vi "AMB_Control.vi"(0 "ObjHandle in":u32, 1 "Data in":u8[](array[numeric]) format="%.0x", 2 "CAN ID in":u32 format="%.0x", 3 "error in":errorcluster {"code" format="%.0x"}, 4 "Data Length in":u8) -> (5 "ObjHandle out":u32, 6 "error out":errorcluster {"code" format="%.0x"})   [LabVIEW 2017]
doc: "ALMA M&C Bus transmit control message\nTransmits a CAN message to the specified ID.\nreally its just a wrapper for the NICAN WriteNet vi."
panel:
  # "ALMA Monitor and Control Bus\nTransmit Control Message"
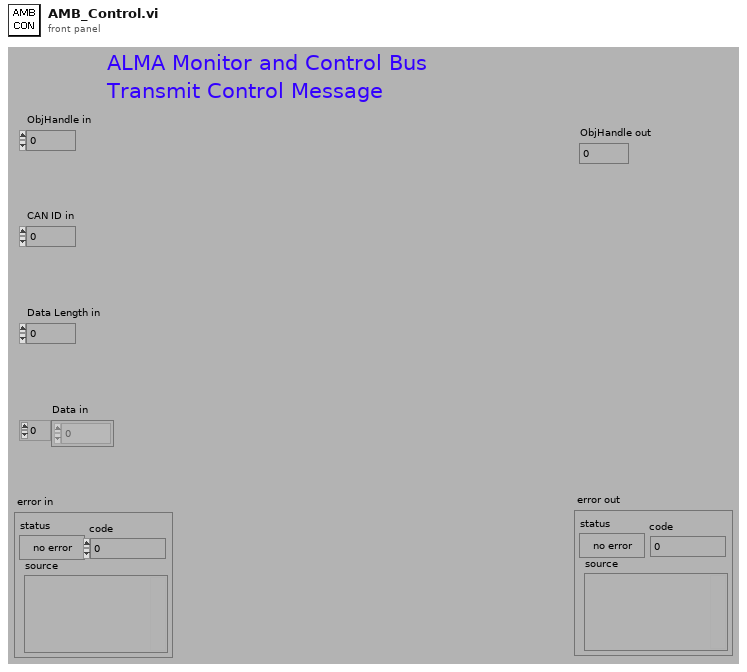
[diagram p1: front panel]
types:
  T1 = typedef "xobjhandle.ctl" = u32
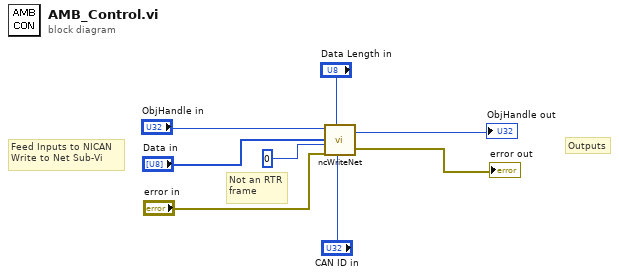
[diagram p0: block diagram]
diagram:
  # "Outputs"
  # "Not an RTR\nframe"
  # "Feed Inputs to NICAN\nWrite to Net Sub-Vi"
  n1 = call <vilib>:"ncWriteNet.vi"("ArbitrationId"="CAN ID in", "DataLength"="Data Length in", "Error in"="error in", "IsRemote"=u8 0, "Data"="Data in", "ObjHandle in"="ObjHandle in") -> ("Error out"=→"error out":errorcluster, "ObjHandle out"=→"ObjHandle out":T1)
